vi "SW_Gen_Available_TTL_outputs_array.vi"(1 "IO 2 configuration":u16, 2 "IO 1 configuration":u16, 3 "SYNC configuration":u16) -> (0 "Available TTL outputs array":cluster{"String":string, "Value":i32}[](array[cluster]))   [LabVIEW 2016]
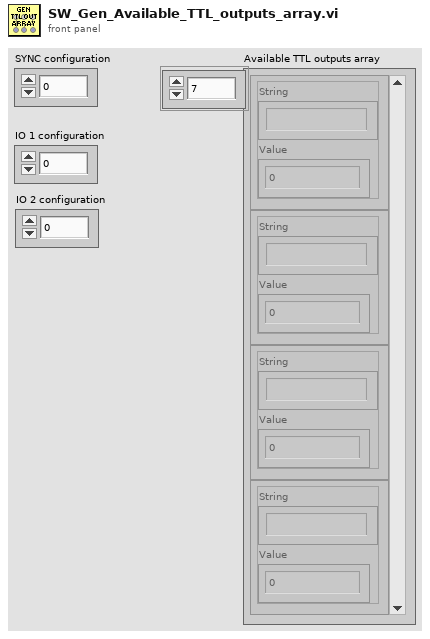
[diagram p1: front panel]
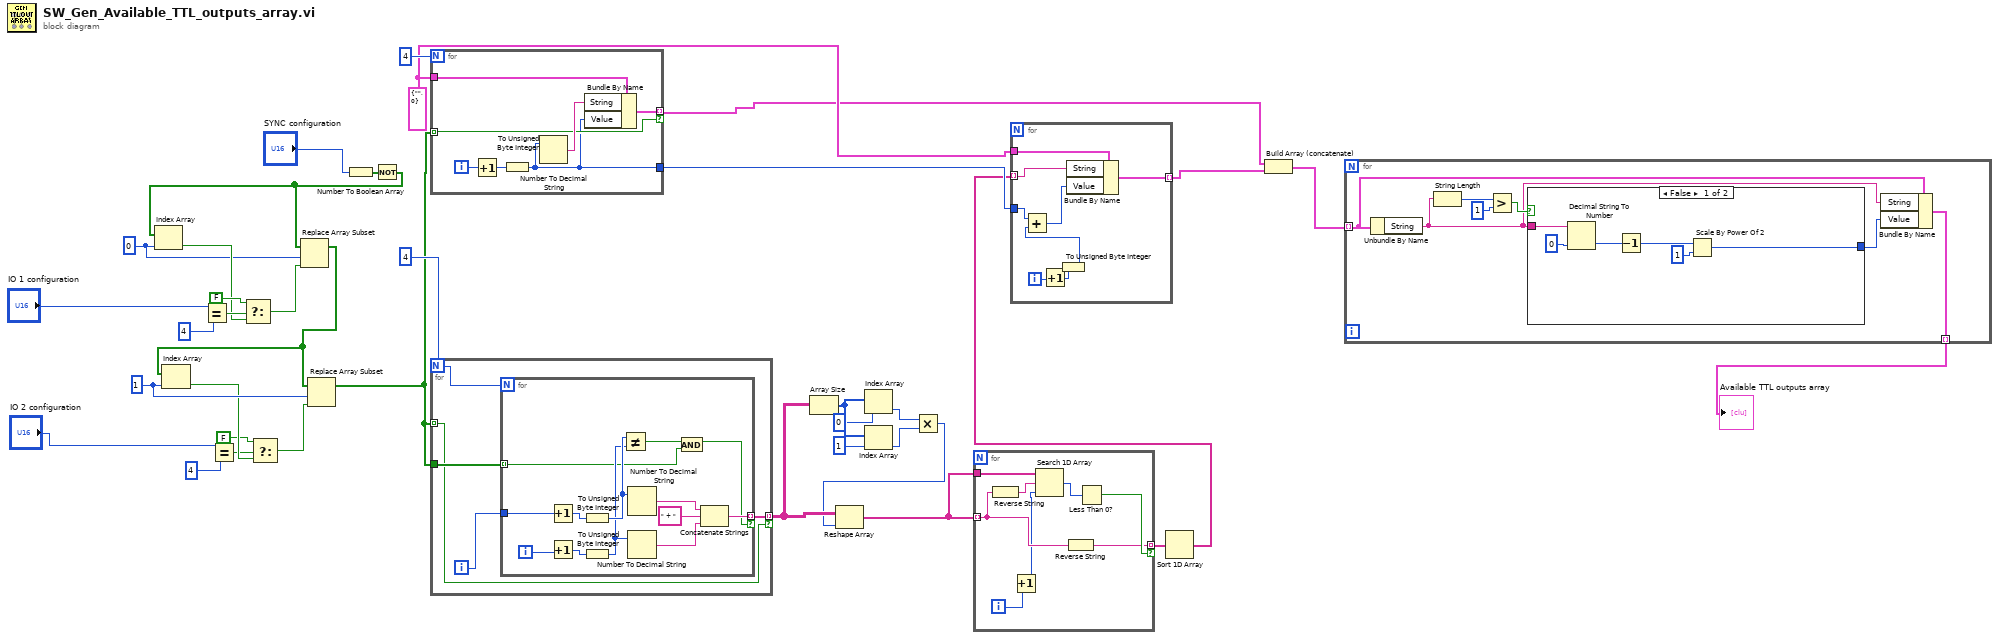
[diagram p0: block diagram]
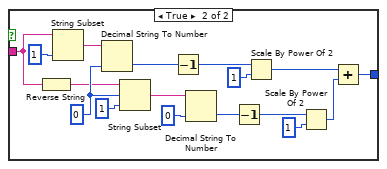
[diagram p2: hidden frame]
diagram:
  w9 = 1 ("index")
  w10 = 0 ("index")
  w24 = cluster{"String":string, "Value":u8} {"String"="", "Value"=0} ("Stim. cluster")
  n1 = Equal?(x="IO 1 configuration", y=u16 4) -> (x = y?=w14:bool)
  n2 = Equal?(x="IO 2 configuration", y=u16 4) -> (x = y?=w5:bool)
  n3 = Number To Boolean Array(number="SYNC configuration") -> (Boolean array=w37:bool[])
  n4 = Not(x=w37) -> (.not. x?=w17:bool[])
  n5 = Index Array(array=w17, index=w10) -> (element=w12:bool)
  n6 = Select(t=FALSE, s=w14, f=w12) -> (s? t:f=w11:bool)
  n7 = Replace Array Subset(array=w17, new element=w11, index=w10) -> (w2:bool[])
  n8 = Index Array(array=w2, index=w9) -> (element=w7:bool)
  n9 = Select(t=FALSE, s=w5, f=w7) -> (s? t:f=w8:bool)
  n10 = Replace Array Subset(array=w2, new element=w8, index=w9) -> (w1:bool[])
  n11 = for {
    N: 4 -> [_]
    tunnel: w1 -> [w39] mode=indexing
    tunnel: w24 -> [w42]
    tunnel: [w40] -> w22 mode=indexing if=w39
    tunnel: [w38] -> w25
    i -> [w44]
    n12 = Increment(x=w44) -> (x+1=w43:i32)
    n13 = To Unsigned Byte Integer(number=w43) -> (unsigned 8bit integer=w38:u8)
    n14 = Number To Decimal String(number=w38) -> (decimal integer string=w41:string)  [unwired: 1 in]
    n15 = Bundle By Name(cluster=w42, "String"=w41, "Value"=w38) -> (w40:cluster{"String":string, "Value":u8})
  }
  n16 = for {
    N: 4 -> [w49]
    tunnel: [w47] -> w33 mode=indexing if=w45
    tunnel: w1 -> [w45] mode=indexing
    tunnel: w1 -> [w46]
    i -> [w48]
    n17 = for {
      N: w49 -> [_]
      tunnel: w48 -> [w61]
      tunnel: [w55] -> w47 mode=indexing if=w51
      tunnel: w46 -> [w50] mode=indexing
      i -> [w62]
      n18 = Increment(x=w61) -> (x+1=w60:i32)
      n19 = Increment(x=w62) -> (x+1=w59:i32)
      n20 = To Unsigned Byte Integer(number=w60) -> (unsigned 8bit integer=w54:u8)
      n21 = To Unsigned Byte Integer(number=w59) -> (unsigned 8bit integer=w53:u8)
      n22 = Not Equal?(x=w54, y=w53) -> (x != y?=w52:bool)
      n23 = Number To Decimal String(number=w54) -> (decimal integer string=w58:string)  [unwired: 1 in]
      n24 = Number To Decimal String(number=w53) -> (decimal integer string=w57:string)  [unwired: 1 in]
      n25 = And(x=w52, y=w50) -> (x .and. y?=w51:bool)
      n26 = Concatenate Strings(w58, " + " ("string"), w57) -> (w55:string)
    }
  }
  n27 = Array Size(array=w33) -> (size(s)=w32:i32[])
  n28 = Index Array(array=w32, index=0) -> (element=w29:i32)
  n29 = Index Array(array=w32, index=1) -> (element=w28:i32)
  n30 = Multiply(x=w29, y=w28) -> (x*y=w27:i32)
  n31 = Reshape Array(w33, w27) -> (w26:string[])
  n32 = for {
    tunnel: w26 -> [w68] mode=indexing
    tunnel: [w63] -> w21 mode=indexing if=w66
    tunnel: w26 -> [w70]
    i -> [w65]
    n33 = Reverse String(1:w68) -> (0:w69:string)
    n34 = Increment(x=w65) -> (x+1=w64:i32)
    n35 = Search 1D Array(1D array=w70, element=w69, start index (0)=w64) -> (index of element=w67:i32)
    n36 = Reverse String(1:w68) -> (0:w63:string)
    n37 = Less Than 0?(x=w67) -> (x < 0?=w66:bool)
  }
  n38 = Sort 1D Array(array=w21) -> (sorted array=w20:string[])
  n39 = for {
    tunnel: w20 -> [w76] mode=indexing
    tunnel: w25 -> [w75]
    tunnel: w24 -> [w77]
    tunnel: [w71] -> w23 mode=indexing
    i -> [w78]
    n40 = Increment(x=w78) -> (x+1=w74:i32)
    n41 = To Unsigned Byte Integer(number=w74) -> (unsigned 8bit integer=w72:u8)
    n42 = Add(x=w75, y=w72) -> (x+y=w73:u8)
    n43 = Bundle By Name(cluster=w77, "String"=w76, "Value"=w73) -> (w71:cluster{"String":string, "Value":u8})
  }
  n44 = Build Array (concatenate)(w22, w23) -> (w19:cluster{"String":string, "Value":u8}[])
  n45 = for {
    tunnel: w19 -> [w82] mode=indexing
    tunnel: [w80] -> w18 mode=indexing
    n46 = Unbundle By Name(w82) -> ("String"=w81:string)
    n47 = String Length(string=w81) -> (length=w85:i32)
    n48 = Greater?(x=w85, y=1) -> (0:w83:bool)
    n49 = case shown="False" w83 {
      tunnel: w81 -> [w91 w102]
      tunnel: [w86 w92] -> w79
      frame False {
        n50 = Decimal String To Number(string=w91, default (0L)=u8 0 ("default (0 I32)")) -> (number=w87:u8)  [unwired: 1 in, 1 out]
        n51 = Decrement(x=w87) -> (x-1=w88:u8)
        n52 = Scale By Power Of 2(n=w88, x=u8 1) -> (x*2^n=w86:u8)
      }
      frame True {
        w103 = u8 0 ("default (0 I32)")
        n53 = Reverse String(1:w102) -> (0:w101:string)
        n54 = String Subset(string=w102, length (rest)=1 ("length (rest)")) -> (substring=w107:string)  [unwired: 1 in]
        n55 = Decimal String To Number(string=w107, default (0L)=w103) -> (number=w100:u8)  [unwired: 1 in, 1 out]
        n56 = String Subset(string=w101, offset (0)=w103, length (rest)=1 ("length (rest)")) -> (substring=w105:string)
        n57 = Decrement(x=w100) -> (x-1=w99:u8)
        n58 = Decimal String To Number(string=w105, default (0L)=u8 0 ("default (0 I32)")) -> (number=w95:u8)  [unwired: 1 in, 1 out]
        n59 = Decrement(x=w95) -> (x-1=w96:u8)
        n60 = Scale By Power Of 2(n=w99, x=u8 1) -> (x*2^n=w94:u8)
        n61 = Scale By Power Of 2(n=w96, x=u8 1) -> (x*2^n=w93:u8)
        n62 = Add(x=w94, y=w93) -> (x+y=w92:u8)
      }
    }
    n63 = Bundle By Name(cluster=w82, "String"=w81, "Value"=w79) -> (w80:cluster{"String":string, "Value":u8})
  }
  "Available TTL outputs array" <- w18
